vi "Write Action.vi"(8 "error in (no error)":errorcluster, 10 "Action":T1=4 items=["Switch when pressed", "Switch when released", "Switch until release", "Latch when pressed", "Latch when released", "Latch until released"], 11 "Control in":refnum<class "Control.lvclass">) -> (0 "error out":errorcluster, 3 "Control out":refnum<class "Control.lvclass">)   [LabVIEW 2013, in "uitools_Control.lvlib" / "Control.lvclass"]
uses:
  Control.lvclass
  Typedefs/TypeDef_Action.ctl
  Control.lvclass/Control.ctl
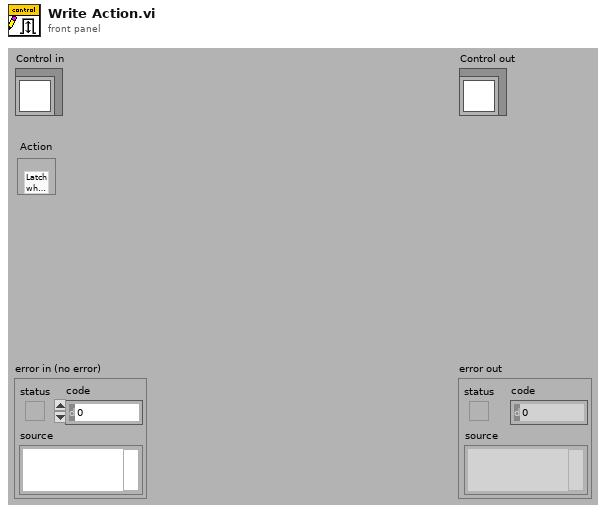
[diagram p1: front panel]
types:
  T1 = typedef "uitools_Control.lvlib/Control.lvclass/TypeDef_Action.ctl" = u16
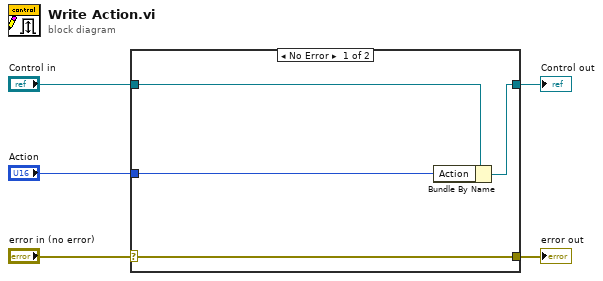
[diagram p0: block diagram]
diagram:
  n1 = case shown="No Error" "error in (no error)" {
    selector: "error in (no error)" -> [w9 w10]
    tunnel: [w9 w10] -> w4
    tunnel: [w7 w11] -> w2
    tunnel: "Control in" -> [w8 w11]
    tunnel: "Action" -> [w6 _]
    frame No Error {
      n2 = Bundle By Name(cluster=w8, "Action"=w6) -> (w7:refnum<class "Control.lvclass">)
    }
    frame Error {
    }
  }
  "error out" <- w4
  "Control out" <- w2
